vi "Set State_Measure SMU_Current_Experiment.vi"(6 "SMU Settings":T2={"Level"=0.01, "Level Range"=0.1, "Limit"=1.0, "Limit Range"=6.0, "Sense"=1009} {"Sense" items=["Local"=1008, "Remote"=1009]}, 7 "script name":string, 8 "error in (no error)":errorcluster, 9 "Published Data Ids":string[](array[string]), 10 "Pins":string[](array[string])=["VDD"], 11 "Semiconductor Module Context":T3) -> (0 "error Out":errorcluster)   [LabVIEW 2013]
uses:
  <vilib>/NI_TestStand_SemiconductorModule/NI_TestStand_Semiconductor_Module.lvlibp/PinMap/General/SemiconductorModuleContext.ctl
  <instrlib>/niDCPower/nidcpower.llb/niDCPower Sense.ctl
  <instrlib>/niHSDIO/niHSDIO.llb/niHSDIO_ctl Trigger Script - trigID Values (Ring).ctl
  <vilib>/NI_TestStand_SemiconductorModule/NI_TestStand_Semiconductor_Module.lvlibp/PinMap/DC Power/PinsToNIDCPowerSessions.vi
  <vilib>/NI_TestStand_SemiconductorModule/NI_TestStand_Semiconductor_Module.lvlibp
panel:
  out "R Array":dbl[][](array[numeric]) format="%#_6p"
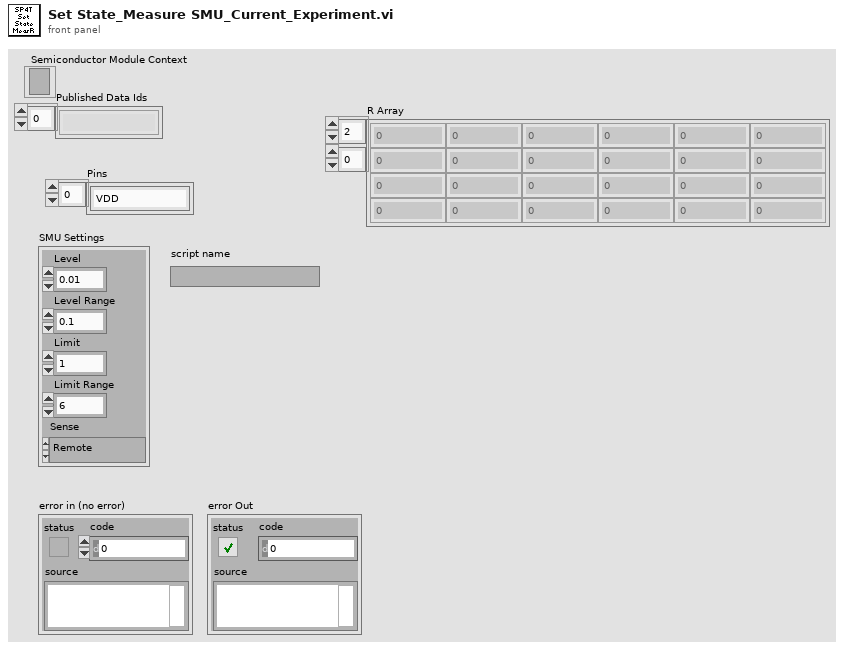
[diagram p1: front panel]
types:
  T1 = typedef "niDCPower Sense.ctl" = i32
  T2 = cluster{"Level":dbl, "Level Range":dbl, "Limit":dbl, "Limit Range":dbl, "Sense":T1}
  T3 = typedef "NI_TestStand_Semiconductor_Module.lvlibp/SemiconductorModuleContext.ctl" = refnum<k7>
  T4 = typedef "niHSDIO_ctl Trigger Script - trigID Values (Ring).ctl" = string
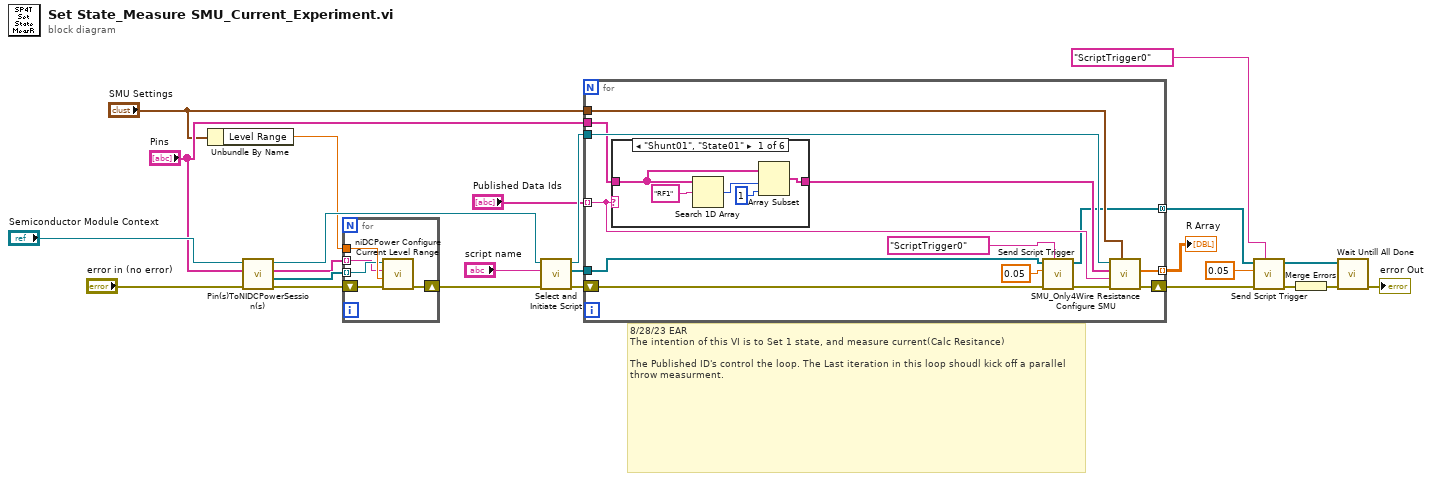
[diagram p0: block diagram]
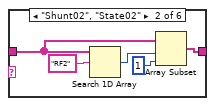
[diagram p2: hidden frame]
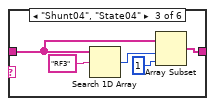
[diagram p3: hidden frame]
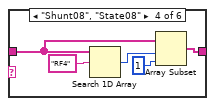
[diagram p4: hidden frame]
diagram:
  # "8/28/23 EAR\nThe intention of this VI is to Set 1 state, and measure current(Calc Resitance)\n\nThe Published ID's control the loop. The Last iteration in this loop shoudl kick off a parallel throw measurment."
  n1 = Unbundle By Name("SMU Settings") -> ("Level Range"=w5:dbl)
  n2 = call-poly <vilib>:"Pin(s)ToNIDCPowerSession(s).vi"("error in (no error)"="error in (no error)", "Pins"="Pins", "Semiconductor Module Context"="Semiconductor Module Context") -> ("error out"=w4:errorcluster, "Instrument Sessions"=w2:refnum<k15>[], "Channel Lists"=w1:string[], "Semiconductor Module Context Out"=w9:T3)  [unwired: 4 in, 1 out]
  n3 = for {
    tunnel: w5 -> [w29]
    shift-right: [w27] -> w3
    shift-left: w4 -> [w28]
    tunnel: w2 -> [w26] mode=indexing
    tunnel: w1 -> [w25] mode=indexing
    n4 = call <instrlib>:"niDCPower Configure Current Level Range.vi"("error in (no error)"=w28, "current level range"=w29, "channel name"=w25, "instrument handle"=w26) -> ("error out"=w27:errorcluster)  [unwired: 6 in, 1 out]
  }
  n5 = call "Select and Initiate Script.vi"("error in (no error)"=w3, "script name"="script name", "Semiconductor Module Context"=w9) -> ("error out"=w24:errorcluster, "HSDIO GEN Sessions Out"=w23:refnum<k15>[], "Semiconductor Module Context Out"=w21:T3)  [unwired: 6 in]
  n6 = for {
    tunnel: w23 -> [w41]
    tunnel: "SMU Settings" -> [w40]
    tunnel: w21 -> [w39]
    tunnel: "Published Data Ids" -> [w33] mode=indexing
    tunnel: "Pins" -> [w35]
    tunnel: [w36] -> w19 mode=indexing
    tunnel: [w32] -> w13 mode=concatenating
    shift-right: [w42] -> w14
    shift-left: w24 -> [w30]
    n7 = case shown="\"Shunt01\", \"State01\"" w33 {
      tunnel: w35 -> [w46 w49 w56 w58 w63 w64]
      tunnel: [w45 w48 w55 w59 w63 w64] -> w34
      frame "Shunt01", "State01" {
        n8 = Search 1D Array(1D array=w46, element="RF1") -> (index of element=w44:i32)  [unwired: 1 in]
        n9 = Array Subset(array=w46, index=w44, length=1) -> (w45:string[])
      }
      frame "Shunt02", "State02" {
        n10 = Search 1D Array(1D array=w49, element="RF2") -> (index of element=w51:i32)  [unwired: 1 in]
        n11 = Array Subset(array=w49, index=w51, length=1) -> (w48:string[])
      }
      frame "Shunt04", "State04" {
        n12 = Search 1D Array(1D array=w56, element="RF3") -> (index of element=w54:i32)  [unwired: 1 in]
        n13 = Array Subset(array=w56, index=w54, length=1) -> (w55:string[])
      }
      frame "Shunt08", "State08" {
        n14 = Search 1D Array(1D array=w58, element="RF4") -> (index of element=w61:i32)  [unwired: 1 in]
        n15 = Array Subset(array=w58, index=w61, length=1) -> (w59:string[])
      }
      frame "Shunt15", "State15" {
      }
      frame "Shunt00", "State00", Default {
      }
    }
    n16 = call "Send Script Trigger.vi"("trigger id (script trigger 0)"=T4 "ScriptTrigger0", "error in (no error)"=w30, "Delay Time (s)"=0.05, "HSDIO Sessions In"=w41) -> ("error out"=w37:errorcluster, "HSDIO Sessions Out"=w32:refnum<k15>[])  [unwired: 6 in]
    n17 = call "SMU_Only4Wire Resistance Configure SMU.vi"("SMU Settings"=w40, "error in (no error)"=w37, "Published Data Id"=w33, "Pins"=w34, "Semiconductor Module Context"=w39) -> ("error Out"=w42:errorcluster, "R Array"=w36:dbl[])  [unwired: 4 in, 1 out]
  }
  "R Array" <- w19
  n18 = call "Send Script Trigger.vi"("trigger id (script trigger 0)"=T4 "ScriptTrigger0", "error in (no error)"=w14, "Delay Time (s)"=0.05, "HSDIO Sessions In"=w13) -> ("error out"=w15:errorcluster, "HSDIO Sessions Out"=w12:refnum<k15>[])  [unwired: 6 in]
  n19 = Merge Errors(w15) -> (w18:errorcluster)
  n20 = call "Wait Untill All Done.vi"("error in (no error)"=w18, "HSDIO Sessions In"=w12) -> ("error out"=→"error Out":errorcluster)  [unwired: 8 in, 1 out]
